vi "Analyze Core.vi"(8 "Error In":errorcluster, 10 "LHW-DataCollection in":refnum<class "LHW-DataCollection.lvclass">, 11 "LHW-Wfm-Analysis-Actor in":refnum<class "LHW-Wfm-Analysis-Actor.lvclass">) -> (0 "Error Out":errorcluster, 2 "LHW-DataCollection out":refnum<class "LHW-DataCollection.lvclass">, 3 "LHW-Wfm-Analysis-Actor out":refnum<class "LHW-Wfm-Analysis-Actor.lvclass">)   [LabVIEW 2016, in "LHW-Wfm-Analysis.lvlib" / "LHW-Wfm-Analysis-Actor.lvclass"]
doc: "Analyze received LHW-DataCollection, append result and update caller."
uses:
  LHW-Wfm-Analysis-Actor.lvclass
  Classes/LHW-Data/LHW-DataCollection/LHW-DataCollection.lvclass
  Classes/LHW-Data/LHW-WfmData/LHW-WfmData.lvclass
  Classes/LHW-Data/LHW-DataCollection/LHW-DataCollection.lvclass/LHW-DataCollection.ctl
  Classes/LHW-Data/LHW-WfmData/LHW-WfmData.lvclass/LHW-WfmData.ctl
  Classes/LHW-Data/LHW-WfmBasicProperties/LHW-WfmBasicProperties.lvclass
  C:/User/Brand/LVP/AF-HelloWorld/Classes/LHW-Data/LHW-Data/LHW-Data.lvclass
  Classes/LHW-Data/LHW-WfmBasicProperties/LHW-WfmBasicProperties.lvclass/LHW-WfmBasicProperties.ctl
  Classes/LHW-Data/LHW-Data/LHW-Data.lvclass/LHW-Data.ctl
  Classes/LHW-Data/LHW-Data/LHW-Data.lvclass
  <vilib>/measure/madcrms.llb/Basic Averaged DC-RMS for 1 Chan.vi
  <vilib>/measure/NI_MAPro.lvlib
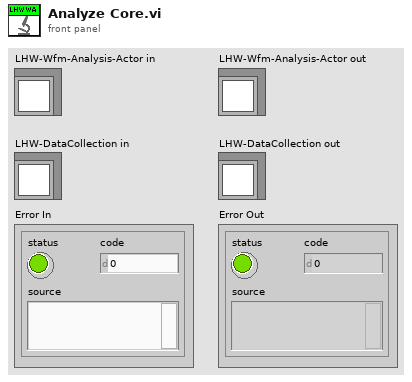
[diagram p1: front panel]
types:
  T1 = enum16{"Rectangular (none)", "Hanning", "Low side lobe"}
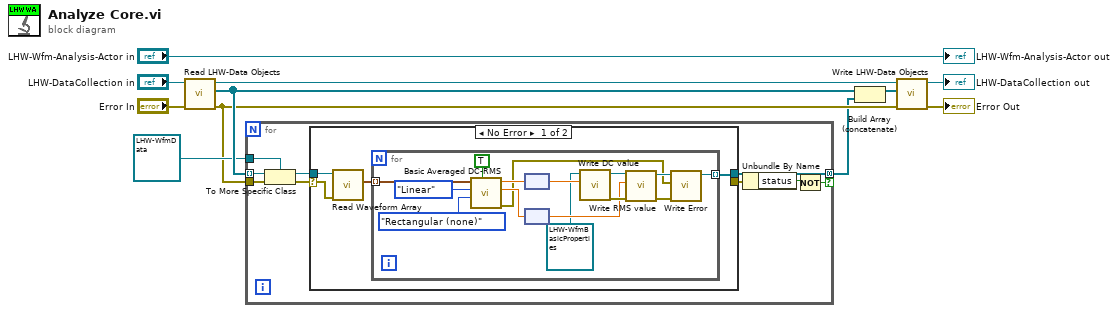
[diagram p0: block diagram]
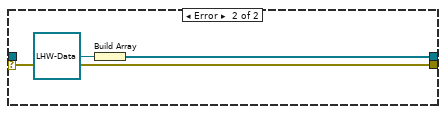
[diagram p2: hidden frame]
diagram:
  n1 = call "Read LHW-Data Objects.vi"("error in (no error)"="Error In", "LHW-DataCollection in"="LHW-DataCollection in") -> ("error out"=w2:errorcluster, "LHW-Data Objects"=w4:refnum<class "LHW-Data.lvclass">[], "LHW-DataCollection out"=w11:refnum<class "LHW-DataCollection.lvclass">)  [unwired: 7 in]
  n2 = for {
    tunnel: w4 -> [w20] mode=indexing
    tunnel: refnum<class "LHW-WfmData.lvclass"> refnum ("LHW-Data.lvlib:LHW-WfmData.lvclass") -> [w19]
    tunnel: w2 -> [w18]
    tunnel: [w15] -> w1 mode=concatenating if=w12
    n3 = To More Specific Class(target class=w19, reference=w20, error in=w18) -> (specific class reference=w16:refnum<class "LHW-WfmData.lvclass">, error out=w17:errorcluster)
    n4 = case shown="No Error" w17 {
      selector: w17 -> [w24 w41]
      tunnel: w16 -> [w23 _]
      tunnel: [w21 w40] -> w15
      tunnel: [_ w41] -> w14
      frame No Error {
        n5 = call "Read Waveform Array.vi"("error in (no error)"=w24, "LHW-WfmData in"=w23) -> ("Waveform Array"=w22:waveform(dbl)[])  [unwired: 7 in, 2 out]
        n6 = for {
          tunnel: w22 -> [w39] mode=indexing
          tunnel: [w27] -> w21 mode=indexing
          n7 = call-poly <vilib>:"Basic Averaged DC-RMS.vi"("reset"=TRUE, "window"=T1."Rectangular (none)", "averaging type"=enum16{"Linear", "Exponential"}."Linear", "signal in"=w39) -> ("error out"=w26:errorcluster, "RMS value"=w33:dbl, "DC value"=w34:dbl)  [unwired: 4 in, 1 out]
          n8 = node(w34) -> (w35:dbl[unit])
          n9 = node(w33) -> (w30:dbl[unit])
          n10 = call "Write DC value.vi"("DC value"=w35, "LHW-WfmBasicProperties in"=refnum<class "LHW-WfmBasicProperties.lvclass"> refnum ("LHW-Data.lvlib:LHW-WfmBasicProperties.lvclass")) -> ("error out"=w31:errorcluster, "LHW-WfmBasicProperties out"=w32:refnum<class "LHW-WfmBasicProperties.lvclass">)  [unwired: 8 in]
          n11 = call "Write RMS value.vi"("error in (no error)"=w31, "RMS value"=w30, "LHW-WfmBasicProperties in"=w32) -> ("error out"=w25:errorcluster, "LHW-WfmBasicProperties out"=w28:refnum<class "LHW-WfmBasicProperties.lvclass">)  [unwired: 7 in]
          n12 = call "Write Error.vi"("error in (no error)"=w25, "Error"=w26, "LHW-Data in"=w28) -> ("LHW-Data out"=w27:refnum<class "LHW-WfmBasicProperties.lvclass">)  [unwired: 7 in, 1 out]
        }
      }
      frame Error {
        n13 = Build Array(refnum<class "LHW-Data.lvclass"> refnum ("LHW-Data.lvlib:LHW-Data.lvclass")) -> (w40:refnum<class "LHW-Data.lvclass">[])
      }
    }
    n14 = Unbundle By Name(w14) -> ("status"=w13:bool)
    n15 = Not(x=w13) -> (.not. x?=w12:bool)
  }
  n16 = Build Array (concatenate)(w4, w1) -> (w10:refnum<class "LHW-Data.lvclass">[])
  n17 = call "Write LHW-Data Objects.vi"("error in (no error)"=w2, "LHW-Data Objects"=w10, "LHW-DataCollection in"=w11) -> ("error out"=→"Error Out":errorcluster, "LHW-DataCollection out"=→"LHW-DataCollection out":refnum<class "LHW-DataCollection.lvclass">)  [unwired: 7 in]
  "LHW-Wfm-Analysis-Actor out" <- "LHW-Wfm-Analysis-Actor in"
